vi "output.vi"(8 "error in":errorcluster, 10 "data table in":T1, 11 "Tagbus PID Module runtime in":refnum<class "Tagbus PID Module runtime.lvclass">) -> (0 "error out":errorcluster, 2 "data table out":T1, 3 "Tagbus PID Module runtime out":refnum<class "Tagbus PID Module runtime.lvclass">)   [LabVIEW 2014, in "Tagbus PID Module runtime.lvclass"]
doc: "Provides an interface for writing data to a module at runtime. While this interface performs no operations, a child should provide an override which may write to any open sessions, references, or interfaces."
uses:
  Tagbus PID Module runtime.lvclass
  <vilib>/NI/Tag Bus/table/data table.ctl
  Tagbus PID Module runtime.lvclass/Tagbus PID Module runtime.ctl
  <vilib>/NI/Tag Bus/table/data polymorphs/read many/read Doubles.vi
  <vilib>/NI/Tag Bus/table/data table.lvlib
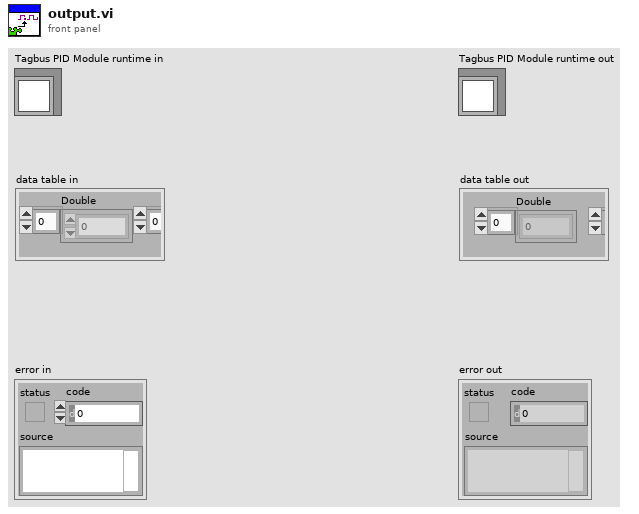
[diagram p1: front panel]
types:
  T1 = typedef "tag bus.lvlib/data table.lvlib/data table.ctl" = cluster{"Double":dbl[], "Single":sgl[], "I64":i64[], "I32":i32[], "I16":i16[], "I8":i8[], "U64":u64[], "U32":u32[], "U16":u16[], "U8":u8[], "Boolean":bool[], "String":string[], "Array of Double":cluster{"DBL Array":dbl[]}[], "Array of Single":cluster{"SGL Array":sgl[]}[], "Array of I64":cluster{"I64 Array":i64[]}[], "Array of I32":cluster{"I32 Array":i32[]}[], "Array of I16":cluster{"I16 Array":i16[]}[], "Array of I8":cluster{"I8 Array":i8[]}[], "Array of U64":cluster{"U64 Array":u64[]}[], "Array of U32":cluster{"U32 Array":u32[]}[], "Array of U16":cluster{"U16 Array":u16[]}[], "Array of U8":cluster{"U8 Array":u8[]}[], "Array of Boolean":cluster{"Boolean Array":bool[]}[], "Array of String":cluster{"String Array":string[]}[]}
  T2 = cluster{"control indices":i32[], "data indices":i32[]}[]
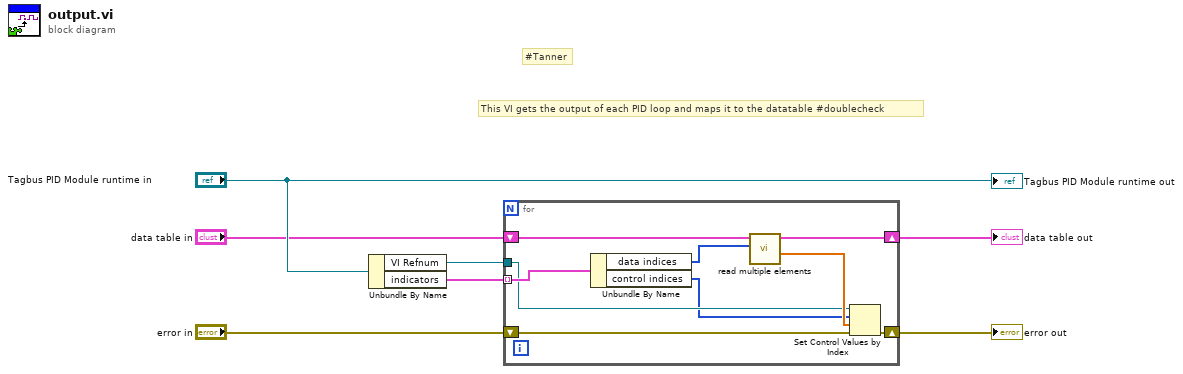
[diagram p0: block diagram]
diagram:
  # "#Tanner"
  # "This VI gets the output of each PID loop and maps it to the datatable #doublecheck"
  n1 = Unbundle By Name("Tagbus PID Module runtime in") -> ("VI Refnum"=w6:refnum<vi>, "indicators"=w5:T2)
  n2 = for {
    tunnel: w6 -> [w11]
    tunnel: w5 -> [w16] mode=indexing
    shift-right: [w14] -> w3
    shift-left: "data table in" -> [w15]
    shift-right: [w8] -> w1
    shift-left: "error in" -> [w9]
    n3 = Unbundle By Name(w16) -> ("data indices"=w13:i32[], "control indices"=w10:i32[])
    n4 = call-poly <vilib>:"read multiple elements.vi"("indices"=w13, "data table in"=w15) -> ("values"=w12:dbl[], "data table out"=w14:T1)  [unwired: 8 in]
    n5 = Set Control Values by Index(0:w11, 1:w10, 2:w12, 3:w9) -> (11:w8:errorcluster)
  }
  "error out" <- w1
  "data table out" <- w3
  "Tagbus PID Module runtime out" <- "Tagbus PID Module runtime in"
